vi "HovaCAL fixed Komponents.vi"() -> (2 "MFV Komponente fix out":u16[](array[numeric]), 3 "HovaCAL fixed":bool)   [LabVIEW 2020, in "Linearisierung v2.lvlib" / "SpanEinstellungen.lvlib"]
uses:
  SpanEinstellungen.lvlib
  Gasteiler/Aktionen FGV Gasteiler Daten.ctl
  GasteilerType.ctl
  Gasteiler/HovaCAL_Interface/Kommunikation/Aktion FGV HovaCAL Interface Autolin.ctl
  Gasteiler/HovaCAL_Interface/Kommunikation/Kommunikation.lvlib
  Gasteiler/Gasteiler.lvlib
  Linearisierung v2.lvlib
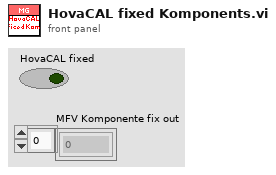
[diagram p1: front panel]
types:
  T1 = typedef "Linearisierung v2.lvlib/GasteilerType.ctl" = u16
  T2 = typedef "Linearisierung v2.lvlib/Gasteiler.lvlib/Aktionen FGV Gasteiler Daten.ctl" = enum16{"lesen", "Gasteiler Daten", "Seriellen Param.", "MB-Endwert", "laden", "speichern", "Anforderung", "TCP", "Aufzeichnung Start"}
  T3 = typedef "Linearisierung v2.lvlib/Gasteiler.lvlib/HovaCAL_Interface.lvlib/Kommunikation.lvlib/Aktion FGV HovaCAL Interface Autolin.ctl" = enum16{"lesen", "schreiben", "MFC Komponente fix setzen", "init"}
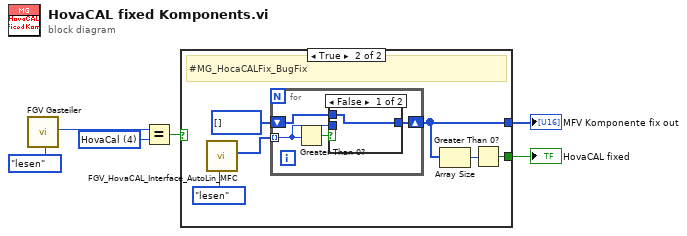
[diagram p0: block diagram]
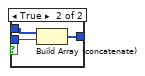
[diagram p3: hidden frame]
diagram:
  w4 = T1 4 items=["LNI", "Analog-Display", "AVL GDU", "Horiba GDC", "HovaCal", "Horiba SGD 710C"] ("y")
  n1 = call "FGV Gasteiler.vi"("Aktionen"=Aktionen_FGV_Gasteiler_Daten."lesen") -> ("Gasteiler Type"=w5:T1)  [unwired: 11 in, 7 out]
  n2 = Equal?(x=w5, y=w4) -> (x = y?=w2:bool)
  n3 = case shown="True" w2 {
    tunnel: [_ w10] -> w3
    tunnel: [_ w7] -> w1
    frame False {
    }
    frame True {
      # "#MG_HocaCALFix_BugFix"
      n4 = call "FGV_HovaCAL_Interface_AutoLin_MFC.vi"("Aktion"=Aktion_FGV_HovaCAL_Interface_Autolin."lesen") -> ("MFV Komponente fix out"=w9:u16[])  [unwired: 7 in, 3 out]
      n5 = for {
        tunnel: w9 -> [w15] mode=indexing
        shift-right: [w14] -> w7
        shift-left: u16[] [] -> [w13]
        n6 = Greater Than 0?(x=w15) -> (x > 0?=w16:bool)
        n7 = case shown="False" w16 {
          tunnel: w15 -> [_ w20]
          tunnel: [w17 w19] -> w14
          tunnel: w13 -> [w17 w18]
          frame False {
          }
          frame True {
            n8 = Build Array (concatenate)(w18, w20) -> (w19:u16[])
          }
        }
      }
      n9 = Array Size(array=w7) -> (size(s)=w11:i32)
      n10 = Greater Than 0?(x=w11) -> (x > 0?=w10:bool)
    }
  }
  "HovaCAL fixed" <- w3
  "MFV Komponente fix out" <- w1
